vi "Measure Channel.vi"(7 "Measurement Type":T1, 8 "error in (no error)":errorcluster, 9 "Channel":string, 10 "Instrument":string, 11 "Driver Test in":refnum<class "Driver Test.lvclass">) -> (0 "error out":errorcluster, 2 "Additional Info":variant, 3 "Measurement":dbl)   [LabVIEW 2015, in "Driver Test.lvclass"]
uses:
  Driver Test.lvclass
  Measurement Type -- Enum.ctl
  CBTF Applications/Driver Board Testing/Main/Application/Application/Class/typedefs/Instrument Selector -- Enum.ctl
  Classes/Instruments/Digital Power Meter/Digital Power Meter/Class/Digital Power Meter.lvclass
  Classes/Instruments/MIO Device/DAQmx Device/Class/DAQmx Device.lvclass
  Classes/Instruments/MIO Device/MIO Device/Class/typedefs/Read Type -- Enum.ctl
  Classes/Instruments/MIO Device/MIO Device/Class/typedefs/Channel Type -- Enum.ctl
  Classes/Instruments/MIO Device/MIO Device/Class/typedefs/Channel Configuration -- Cluster.ctl
  Classes/Instruments/Power Supply/Class/Power Supply.lvclass
  CBTF Applications/Driver Board Testing/Main/Application/Application/Class/Driver Board Test.lvclass
  Classes/Instruments/MIO Device/MIO Device/Class/MIO Device.lvclass
  Test Class/Test Class.lvclass
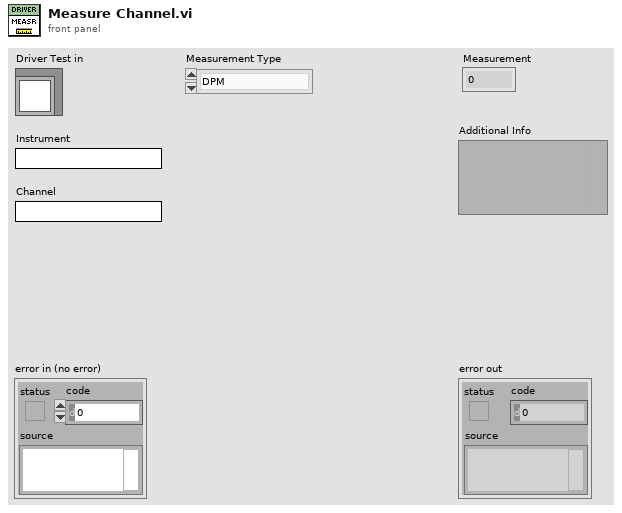
[diagram p1: front panel]
types:
  T1 = typedef "Driver Test.lvclass/Measurement Type -- Enum.ctl" = enum16{"DPM", "DAQmx", "ACPS Voltage", "ACPS Current", "ACPS Power", "DCPS Voltage", "DCPS Current", "DCPS Power"}
  T2 = typedef "Driver Board Test.lvlib/Driver Board Test.lvclass/Instrument Selector -- Enum.ctl" = enum16{"ACPS1", "ACPS2", "DCPS1", "DCPS2", "DCPS3", "DCLoad1", "DCLoad2", "DPM1", "DPM2", "Switch1", "PXI1Slot2", "PXI1Slot3", "cDAQ1Mod5", "cDAQ1Mod6", "cDAQ1Mod7", "cDAQ1Mod8", "cDAQ1Mod1", "cDAQ1Mod2", "cDAQ1Mod3", "cDAQ1Mod4", "cDAQ2Mod1", "cDAQ2Mod2", "cDAQ2Mod3", "cDAQ2Mod4"}
  T3 = typedef "MIO Device.lvlib/MIO Device.lvclass/Channel Configuration -- Cluster.ctl" = cluster{"AI Sample Speed":dbl, "Analog Input Channels":cluster{"Voltage Minimum":dbl, "Voltage Maximum":dbl}[], "Analog Output Channels":cluster{"Voltage Minimum":dbl, "Voltage Maximum":dbl}[], "Digital Channels":cluster{"Output":bool, "Open Collector":bool}[]}
  T4 = typedef "MIO Device.lvlib/MIO Device.lvclass/Channel Type -- Enum.ctl" = enum16{"Analog Input", "Analog Output", "Digital Input", "Digital Output"}
  T5 = typedef "MIO Device.lvlib/MIO Device.lvclass/Read Type -- Enum.ctl" = enum16{"Get All", "Get Latest", "Get Average"}
  T6 = enum16{"Voltage RMS", "Voltage DC", "AC Current", "DC Current", "Frequency", "Real Power", "Reactive Power", "Apparent Power", "Power Factor"}
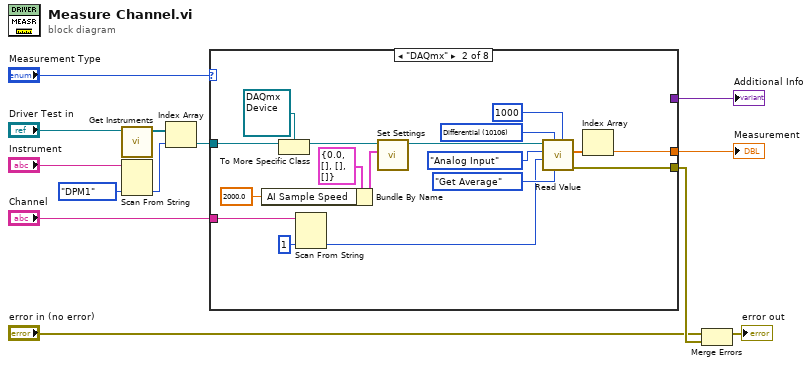
[diagram p0: block diagram]
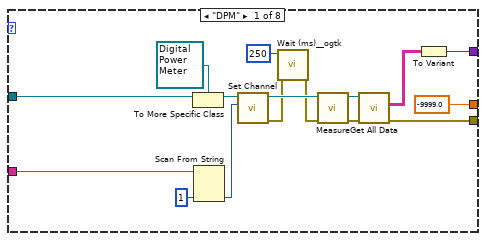
[diagram p2: hidden frame]
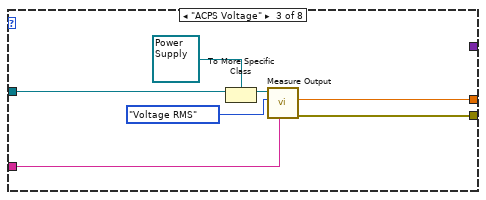
[diagram p3: hidden frame]
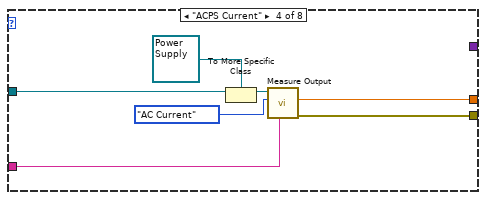
[diagram p4: hidden frame]
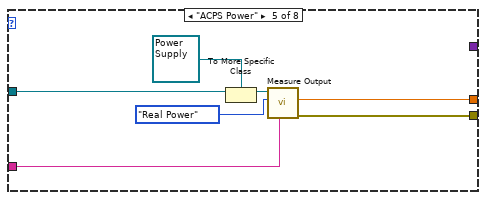
[diagram p5: hidden frame]
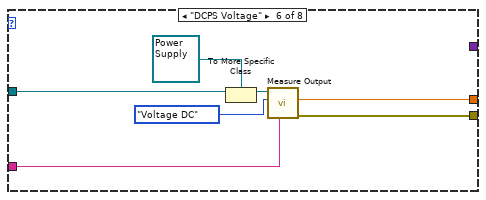
[diagram p6: hidden frame]
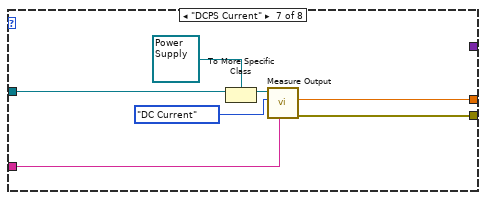
[diagram p7: hidden frame]
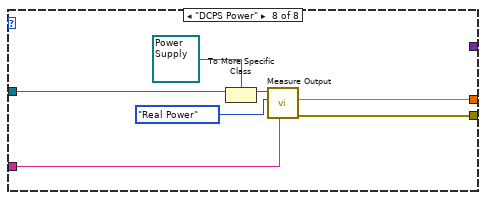
[diagram p8: hidden frame]
diagram:
  n1 = call "Get Instruments.vi"("Test Class in"="Driver Test in") -> ("Instruments"=w1:refnum<class "Instrument.lvclass">[])  [unwired: 9 in, 1 out]
  n2 = Scan From String(input string="Instrument", default 1=Instrument_Selector_--_Enum."DPM1" ("Instrument")) -> (output 1=w12:T2)  [unwired: 3 in, 3 out]
  n3 = Index Array(array=w1, index=w12) -> (element=w11:refnum<class "Instrument.lvclass">)
  n4 = case shown="\"DAQmx\"" "Measurement Type" {
    tunnel: w11 -> [w24 w35 w50 w57 w64 w71 w78 w85]
    tunnel: [-9999.0 ("Measurement") w34 w49 w56 w63 w70 w77 w84] -> w9
    tunnel: [w16 w33 w48 w55 w62 w69 w76 w83] -> w8
    tunnel: "Channel" -> [w14 w31 w47 w54 w61 w68 w75 w82]
    tunnel: [w17 _ _ _ _ _ _ _] -> w3
    frame "DPM" {
      n5 = To More Specific Class(target class=refnum<class "Digital Power Meter.lvclass"> refnum ("Digital Power Meter.lvlib:Digital Power Meter.lvclass"), reference=w24) -> (specific class reference=w28:refnum<class "Digital Power Meter.lvclass">)  [unwired: 1 in, 1 out]
      n6 = Scan From String(input string=w14, default 1=u32 1 ("Channel")) -> (output 1=w21:u32)  [unwired: 3 in, 3 out]
      n7 = call-dynamic "Set Channel.vi"("Channel"=w21, "Acrobat Template in"=w28) -> ("error out"=w26:errorcluster, "Acrobat Template out"=w29:refnum<class "Digital Power Meter.lvclass">)  [unwired: 8 in]
      n8 = call <userlib>:"Wait (ms)__ogtk.vi"("error in (no error)"=w26, "milliseconds to wait"=u32 250) -> ("error out"=w27:errorcluster)  [unwired: 8 in, 1 out]
      n9 = call-dynamic "Measure.vi"("error in (no error)"=w27, "Acrobat Template in"=w29) -> ("error out"=w19:errorcluster, "Acrobat Template out"=w20:refnum<class "Digital Power Meter.lvclass">)  [unwired: 8 in]
      n10 = call "Get All Data.vi"("error in (no error)"=w19, "Acrobat Template in"=w20) -> ("error out"=w16:errorcluster, "Data"=w18:string[][])  [unwired: 7 in, 1 out]
      n11 = To Variant(anything=w18) -> (Variant=w17:variant)
    }
    frame "DAQmx" {
      w39 = 10106 items=["Default"=-1, "RSE"=10083, "NRSE"=10078, "Differential"=10106, "Pseudodifferential"=12529] ("Terminal Config (RSE)")
      n12 = Bundle By Name(cluster=T3 {"AI Sample Speed"=0.0, "Analog Input Channels"=[], "Analog Output Channels"=[], "Digital Channels"=[]} ("Configuration"), "AI Sample Speed"=2000.0) -> (w45:T3)
      n13 = To More Specific Class(target class=refnum<class "DAQmx Device.lvclass"> refnum ("DAQmx Device.lvlib:DAQmx Device.lvclass"), reference=w35) -> (specific class reference=w42:refnum<class "DAQmx Device.lvclass">)  [unwired: 1 in, 1 out]
      n14 = Scan From String(input string=w31, default 1=u32 1 ("Channel")) -> (output 1=w30:u32)  [unwired: 3 in, 3 out]
      n15 = call "Set Settings.vi"("Configuration"=w45, "Acrobat Template in"=w42) -> ("Acrobat Template out"=w43:refnum<class "DAQmx Device.lvclass">)  [unwired: 8 in, 1 out]
      n16 = call-dynamic "Read Value.vi"("Samples to Read (50)"=1000, "Read Function (Get All)"=Read_Type_--_Enum."Get Average", "Terminal Config (RSE)"=w39, "Channel (0)"=w30, "Channel Type"=Channel_Type_--_Enum."Analog Input", "DAQmx Device"=w43) -> ("error out"=w33:errorcluster, "First Channel"=w41:dbl[])  [unwired: 2 in, 2 out]
      n17 = Index Array(array=w41) -> (element=w34:dbl)  [unwired: 1 in]
    }
    frame "ACPS Voltage" {
      n18 = To More Specific Class(target class=refnum<class "Power Supply.lvclass"> refnum ("Power Supply.lvlib:Power Supply.lvclass"), reference=w50) -> (specific class reference=w52:refnum<class "Power Supply.lvclass">)  [unwired: 1 in, 1 out]
      n19 = call-dynamic "Measure Output.vi"("Channel (\"1\")"=w47, "Measurement Type (0: Voltage RMS)"=T6."Voltage RMS", "Acrobat Template in"=w52) -> ("error out"=w48:errorcluster, "Measurement"=w49:dbl)  [unwired: 6 in, 1 out]
    }
    frame "ACPS Current" {
      n20 = To More Specific Class(target class=refnum<class "Power Supply.lvclass"> refnum ("Power Supply.lvlib:Power Supply.lvclass"), reference=w57) -> (specific class reference=w59:refnum<class "Power Supply.lvclass">)  [unwired: 1 in, 1 out]
      n21 = call-dynamic "Measure Output.vi"("Channel (\"1\")"=w54, "Measurement Type (0: Voltage RMS)"=T6."AC Current", "Acrobat Template in"=w59) -> ("error out"=w55:errorcluster, "Measurement"=w56:dbl)  [unwired: 6 in, 1 out]
    }
    frame "ACPS Power" {
      n22 = To More Specific Class(target class=refnum<class "Power Supply.lvclass"> refnum ("Power Supply.lvlib:Power Supply.lvclass"), reference=w64) -> (specific class reference=w66:refnum<class "Power Supply.lvclass">)  [unwired: 1 in, 1 out]
      n23 = call-dynamic "Measure Output.vi"("Channel (\"1\")"=w61, "Measurement Type (0: Voltage RMS)"=T6."Real Power", "Acrobat Template in"=w66) -> ("error out"=w62:errorcluster, "Measurement"=w63:dbl)  [unwired: 6 in, 1 out]
    }
    frame "DCPS Voltage" {
      n24 = To More Specific Class(target class=refnum<class "Power Supply.lvclass"> refnum ("Power Supply.lvlib:Power Supply.lvclass"), reference=w71) -> (specific class reference=w73:refnum<class "Power Supply.lvclass">)  [unwired: 1 in, 1 out]
      n25 = call-dynamic "Measure Output.vi"("Channel (\"1\")"=w68, "Measurement Type (0: Voltage RMS)"=T6."Voltage DC", "Acrobat Template in"=w73) -> ("error out"=w69:errorcluster, "Measurement"=w70:dbl)  [unwired: 6 in, 1 out]
    }
    frame "DCPS Current" {
      n26 = To More Specific Class(target class=refnum<class "Power Supply.lvclass"> refnum ("Power Supply.lvlib:Power Supply.lvclass"), reference=w78) -> (specific class reference=w80:refnum<class "Power Supply.lvclass">)  [unwired: 1 in, 1 out]
      n27 = call-dynamic "Measure Output.vi"("Channel (\"1\")"=w75, "Measurement Type (0: Voltage RMS)"=T6."DC Current", "Acrobat Template in"=w80) -> ("error out"=w76:errorcluster, "Measurement"=w77:dbl)  [unwired: 6 in, 1 out]
    }
    frame "DCPS Power" {
      n28 = To More Specific Class(target class=refnum<class "Power Supply.lvclass"> refnum ("Power Supply.lvlib:Power Supply.lvclass"), reference=w85) -> (specific class reference=w87:refnum<class "Power Supply.lvclass">)  [unwired: 1 in, 1 out]
      n29 = call-dynamic "Measure Output.vi"("Channel (\"1\")"=w82, "Measurement Type (0: Voltage RMS)"=T6."Real Power", "Acrobat Template in"=w87) -> ("error out"=w83:errorcluster, "Measurement"=w84:dbl)  [unwired: 6 in, 1 out]
    }
  }
  "Additional Info" <- w3
  "Measurement" <- w9
  n30 = Merge Errors("error in (no error)", w8) -> (→"error out":errorcluster)
